vi "initializeStage.vi"(9 "VI Ref":refnum<vi>, 10 "HWSerialNum":i32, 11 "reference":refnum<k7>) -> (3 "reference out":refnum<k7>)   [LabVIEW 2016]
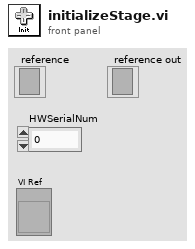
[diagram p1: front panel]
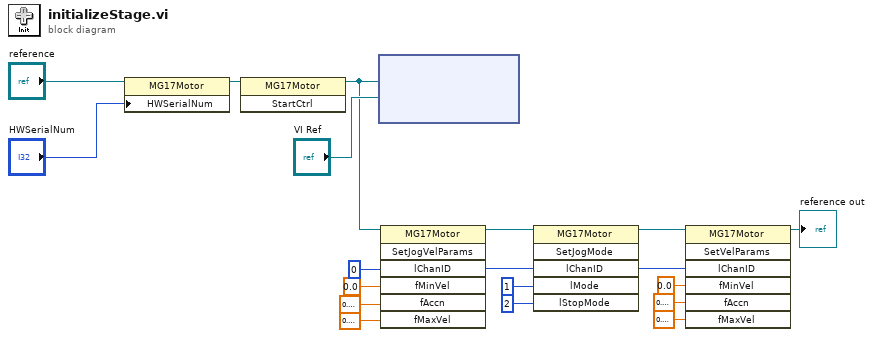
[diagram p0: block diagram]
diagram:
  n1 = property class="MG17Motor"(reference="reference", "HWSerialNum"="HWSerialNum") -> (reference out=w19:refnum<k7>)  [unwired: 1 in, 1 out]
  n2 = invoke class="MG17Motor" method="StartCtrl"(reference=w19) -> (reference out=w2:refnum<k7>)  [unwired: 2 in, 2 out]
  n3 = node(w2, "VI Ref") -> ()  [unwired: 3 in, 2 out]
  n4 = invoke class="MG17Motor" method="SetJogVelParams"(reference=w2, "lChanID"=0, "fMinVel"=sgl 0.0, "fAccn"=sgl 0.4, "fMaxVel"=sgl 0.6) -> (reference out=w9:refnum<k7>, "lChanID"=w8:i32)  [unwired: 2 in, 5 out]
  n5 = invoke class="MG17Motor" method="SetJogMode"(reference=w9, "lChanID"=w8, "lMode"=1 ("plMode"), "lStopMode"=2 ("plStopMode")) -> (reference out=w7:refnum<k7>, "lChanID"=w3:i32)  [unwired: 2 in, 4 out]
  n6 = invoke class="MG17Motor" method="SetVelParams"(reference=w7, "lChanID"=w3, "fMinVel"=sgl 0.0, "fAccn"=sgl 0.4, "fMaxVel"=sgl 0.6) -> (reference out=→"reference out":refnum<k7>)  [unwired: 2 in, 6 out]
